vi "Number GCs.vi"() -> (0 "error out":errorcluster, 1 "Size (um)":u32[](array[numeric])=[50, 50, 50], 2 "No Total Neurons":i32, 3 "Cube out":refnum<class "Grid.lvclass">)   [LabVIEW 2013, in "Grid.lvclass"]
doc: "Set the number of neurons (Mfs, GCs, GOs, PCs, LUs, BAs). If the option is enable (Calculate from densities), use the number of GCs to calculate the other types of neurons according to density ratios in the literature [Solinas et al. 2010]. The order of the Array must correspond with the order of the elements in the type def. Type of Neuron"
uses:
  Grid.lvclass
  Neuron/Neuron.lvclass
  Controls/Neuron Info.ctl
  Controls/Type of Neuron.ctl
  Neuron/Neuron.lvclass/Neuron.ctl
  Grid.lvclass/Grid.ctl
panel:
  in  "Comments":string
  out "Neurons Info Out":T1=[{"N"=0, "Radius"=1.0, "Type"=enum."MF", "Color"=16711680}, {"N"=0, "Radius"=2.0, "Type"=enum."BA", "Color"=16773418}, {"N"=0, "Radius"=4.0, "Type"=enum."GO", "Color"=6618946}, {"N"=0, "Radius"=1.0, "Type"=enum."GC", "Color"=1241087}, {"N"=0, "Radius"=6.0, "Type"=enum."PC", "Color"=16711853}, {"N"=0, "Radius"=1.0, "Type"=enum."LU", "Color"=1114367}]
  in  "Number of GCs":i32
  in  "Cancel Button":bool
  in  "OK Button":bool
  in  "Size Cortex XYZ (um)":dbl[](array[numeric])=[50.0, 50.0, 50.0]
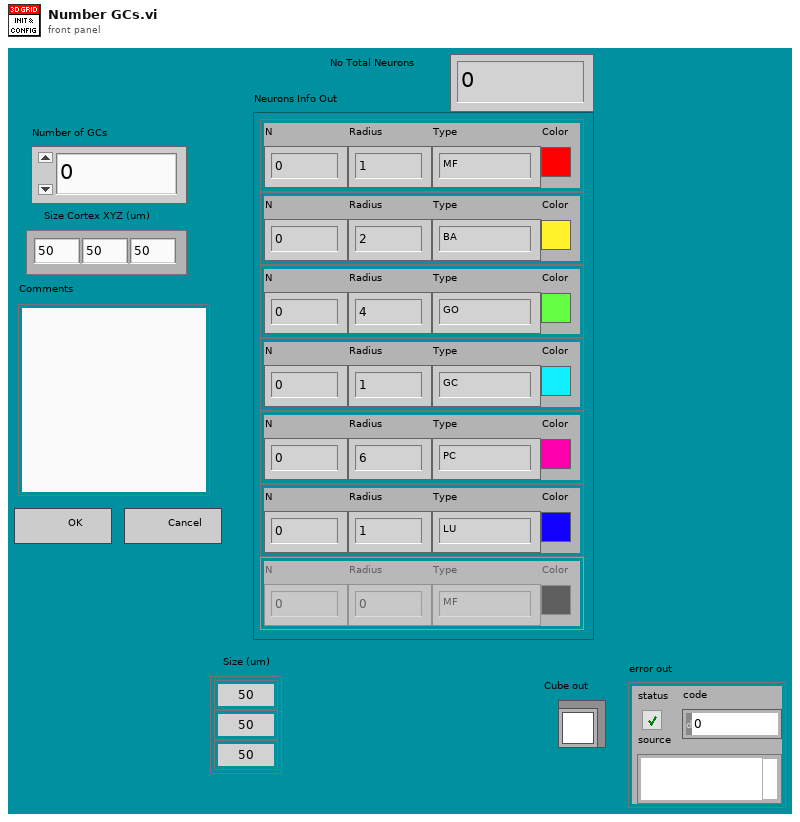
[diagram p1: front panel]
types:
  T1 = typedef "Neuron Info.ctl" = cluster{"N":i32, "Radius":dbl, "Type":T2, "Color":u32}[]
  T2 = typedef "Type of Neuron.ctl" = enum16{"MF", "BA", "GO", "GC", "PC", "LU", "Glia (Dummy)"}
  T3 = cluster{"N":i32, "Radius":dbl, "Type":T2, "Color":u32}
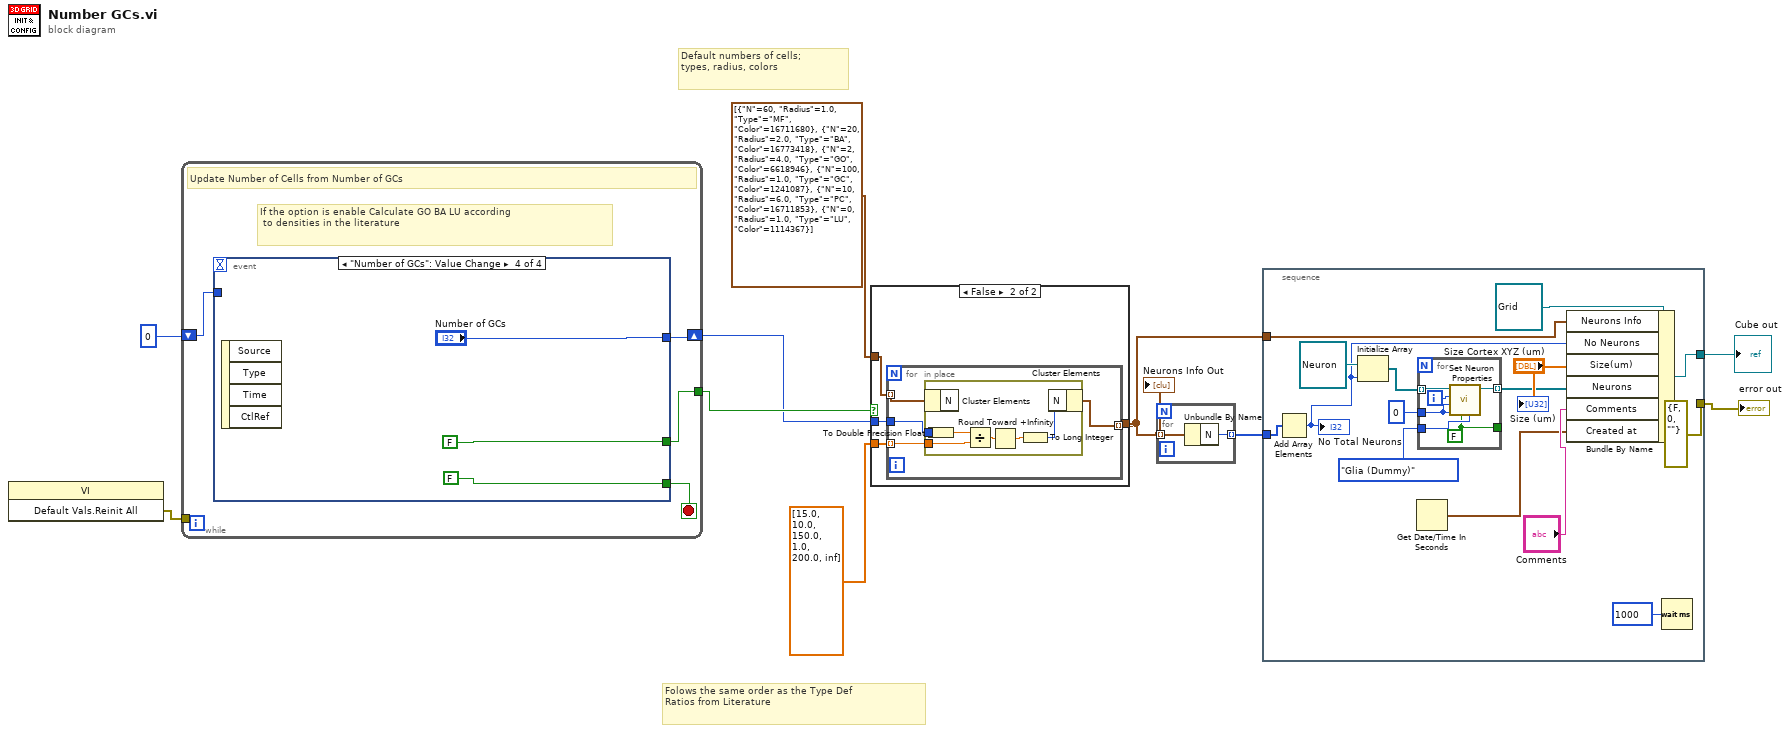
[diagram p0: block diagram]
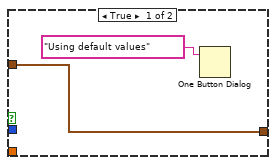
[diagram p2: hidden frame]
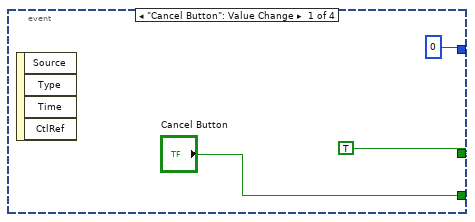
[diagram p3: hidden frame]
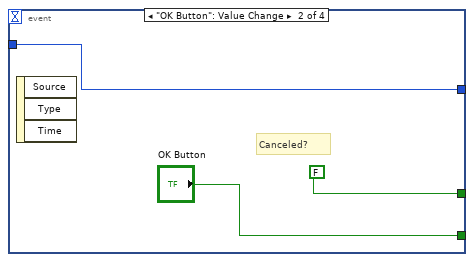
[diagram p4: hidden frame]
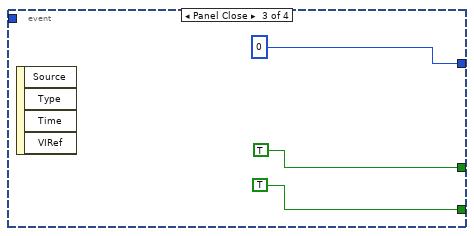
[diagram p5: hidden frame]
diagram:
  # "Default numbers of cells;\ntypes, radius, colors"
  # "Folows the same order as the Type Def\nRatios from Literature"
  n1 = invoke class="VI" method="Default Vals.Reinit All"() -> (error out=w10:errorcluster)  [unwired: 3 in, 2 out]
  n2 = while {
    tunnel: [w13] -> w6
    tunnel: w10 -> [_]
    shift-right: [w11] -> w5
    shift-left: 0 ("N") -> [w12]
    stop <- w14 stop-if-true
    # "If the option is enable Calculate GO BA LU according\n to densities in the literature"
    # "Update Number of Cells from Number of GCs"
    n3 = event shown="[3] \"Number of GCs\": Value Change" {
      selector: _ -> [_ _ _ _]
      dyn-events: _ -> [_ _ _ _]
      timeout: _ -> [_ _ _ _]
      tunnel: ["Cancel Button" "OK Button" TRUE ("OK Button") FALSE ("OK Button")] -> w14
      tunnel: [TRUE ("Cancel Button") FALSE ("Cancel Button") TRUE ("Cancel Button") FALSE ("Cancel Button")] -> w13
      tunnel: [0 ("N") w18 0 ("N") "Number of GCs"] -> w11
      tunnel: w12 -> [_ w18 _ _]
      event "Cancel Button": Value Change {
        n4 = event-data() -> ()  [unwired: 1 in, 4 out]
      }
      event "OK Button": Value Change {
        # "Canceled?"
        n5 = event-data() -> ()  [unwired: 1 in, 3 out]
      }
      event Panel Close {
        n6 = event-data() -> ()  [unwired: 1 in, 4 out]
      }
      event "Number of GCs": Value Change {
        n7 = event-data() -> ()  [unwired: 1 in, 4 out]
      }
    }
  }
  n8 = case shown="False" w6 {
    tunnel: [w28 w32] -> w3
    tunnel: dbl[] [15.0, 10.0, 150.0, 1.0, 200.0, inf] -> [_ w31]
    tunnel: T1 [{"N"=60, "Radius"=1.0, "Type"=enum."MF", "Color"=16711680}, {"N"=20, "Radius"=2.0, "Type"=enum."BA", "Color"=16773418}, {"N"=2, "Radius"=4.0, "Type"=enum."GO", "Color"=6618946}, {"N"=100, "Radius"=1.0, "Type"=enum."GC", "Color"=1241087}, {"N"=10, "Radius"=6.0, "Type"=enum."PC", "Color"=16711853}, {"N"=0, "Radius"=1.0, "Type"=enum."LU", "Color"=1114367}] ("Neurons Info") -> [w28 w30]
    tunnel: w5 -> [_ w29]
    frame True {
      n9 = One Button Dialog(message="Using default values") -> ()  [unwired: 1 in, 1 out]
    }
    frame False {
      n10 = for {
        tunnel: [w36] -> w32 mode=indexing
        tunnel: w31 -> [w35] mode=indexing
        tunnel: w30 -> [w34] mode=indexing
        tunnel: w29 -> [w33]
        n11 = in-place {
          in-place-border: w35 -> [w38]
          in-place-border: w33 -> [w37]
          n12 = in-place-cluster #1(w34) -> ()  [unwired: 1 out]
          n13 = To Double Precision Float(number=w37) -> (double precision float=w42:dbl)
          n14 = Divide(x=w42, y=w38) -> (x/y=w41:dbl)
          n15 = Round Toward +Infinity(x=w41) -> (ceil(x): smallest int >= x=w40:dbl)
          n16 = To Long Integer(number=w40) -> (32bit integer=w39:i32)
          n17 = in-place-cluster #1("N"=w39) -> (w36:T3)
        }
      }
    }
  }
  "Neurons Info Out" <- w3
  n18 = for {
    tunnel: w3 -> [w44] mode=indexing
    tunnel: [w43] -> w2 mode=indexing
    n19 = Unbundle By Name(w44) -> ("N"=w43:i32)
  }
  n20 = stacked-sequence {
    tunnel: [errorcluster {"status"=FALSE, "code"=0, "source"=""} ("error out")] -> w1
    tunnel: [w51] -> w4
    tunnel: w3 -> [w50]
    tunnel: w2 -> [w49]
    frame #0 {
      n21 = Add Array Elements(numeric array=w49) -> (sum=w48:i32)
      "No Total Neurons" <- w48
      n22 = Initialize Array(refnum<class "Neuron.lvclass"> refnum ("CELLUM Neuron.lvclass"), w48) -> (w57:refnum<class "Neuron.lvclass">[])
      n23 = Get Date/Time In Seconds() -> (seconds since 1Jan1904=w45:timestamp)
      n24 = for {
        tunnel: w57 -> [w65] mode=indexing
        tunnel: 0 ("Global ID") -> [w62]
        tunnel: [w64] -> w55 mode=indexing
        tunnel: Type_of_Neuron."Glia (Dummy)" ("Group") -> [w61]
        tunnel: [w60] -> _
        i -> [w63]
        w60 = FALSE ("Active")
        n25 = call "Set Neuron Properties.vi"("Group"=w61, "Active"=w60, "Position Key"=w62, "InGROUP ID"=w62, "ID"=w63, "Neuron in"=w65) -> ("Neuron out"=w64:refnum<class "Neuron.lvclass">)  [unwired: 5 in]
      }
      n26 = Bundle By Name(cluster=refnum<class "Grid.lvclass"> refnum ("CELLUM_Cube in"), "Neurons Info"=w50, "No Neurons"=w48, "Size(um)"="Size Cortex XYZ (um)", "Neurons"=w55, "Comments"="Comments", "Created at"=w45) -> (w51:refnum<class "Grid.lvclass">)
      n27 = Wait (ms)(milliseconds to wait=u32 1000) -> ()  [unwired: 1 out]
      "Size (um)" <- "Size Cortex XYZ (um)"
    }
  }
  "Cube out" <- w4
  "error out" <- w1
